vi "Generate Display Manager DVR.vi"(8 "Error In":errorcluster, 11 "Display Manager In":refnum<class "Display Manager.lvclass">) -> (0 "Error Out":errorcluster, 3 "Display Manager Out":refnum<class "Display Manager.lvclass">)   [LabVIEW 2019, in "Display Manager.lvclass"]
uses:
  Display Manager.lvclass
  Controls/Data.ctl
  <vilib>/Memosfet/myRIO-Neopixel/RT/Display/Display.lvclass
  <vilib>/Memosfet/OpenWeatherAPI/Open Weather Session/Open Weather Session.lvclass
  Display Manager.lvclass/Display Manager.ctl
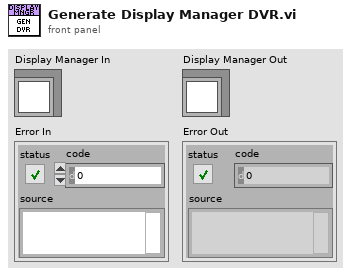
[diagram p1: front panel]
types:
  T1 = typedef "Display Manager.lvclass/Data.ctl" = cluster{"Display":refnum<class "Display.lvclass">, "Open Weather Session":refnum<class "Open Weather Session.lvclass">}
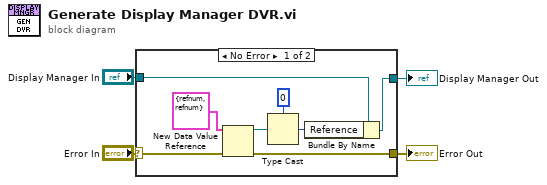
[diagram p0: block diagram]
diagram:
  n1 = case shown="No Error" "Error In" {
    selector: "Error In" -> [w12 w14]
    tunnel: "Display Manager In" -> [w9 w13]
    tunnel: [w8 w13] -> w3
    tunnel: [w7 w14] -> w1
    frame No Error {
      n2 = New Data Value Reference(data value=T1 {"Display"=refnum, "Open Weather Session"=refnum} ("Data"), error in=w12) -> (data value reference=w11:refnum<data-value>, error out=w7:errorcluster)
      n3 = Type Cast(type=u64 0, x=w11) -> (*(type *) &x=w6:u64)
      n4 = Bundle By Name(cluster=w9, "Reference"=w6) -> (w8:refnum<class "Display Manager.lvclass">)
    }
    frame Error {
    }
  }
  "Error Out" <- w1
  "Display Manager Out" <- w3
